vi "Test Get Keys from Map.vi"() -> ()   [LabVIEW 2020]
uses:
  5e20b283-b98d-45fe-82f2-655b53224886.vi
  <vilib>/addons/_JKI Toolkits/Caraya/classes/Assert/Assert Equal Value and Type_Variant.vi
  <vilib>/addons/_JKI Toolkits/Caraya/classes/Test/Test.lvclass
  <vilib>/addons/_JKI Toolkits/Caraya/classes/Assert/Assert.lvclass
panel:
  out "error out":errorcluster
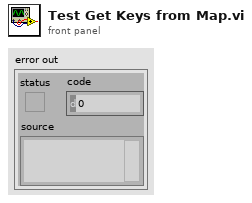
[diagram p1: front panel]
types:
  T1 = cluster{"Name":i32, "value":cluster{"bool":bool, "string":string}}[]
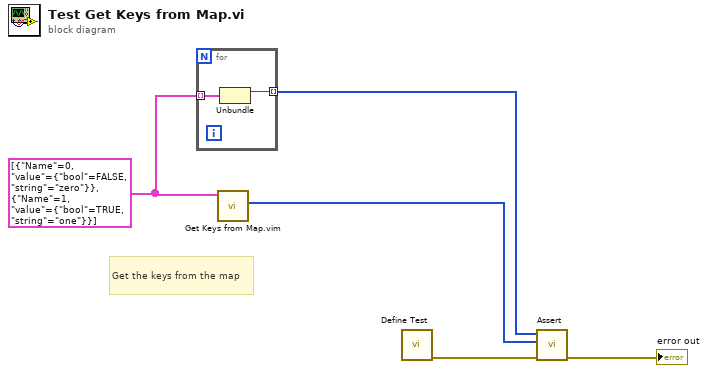
[diagram p0: block diagram]
diagram:
  w2 = T1 [{"Name"=0, "value"={"bool"=FALSE, "string"="zero"}}, {"Name"=1, "value"={"bool"=TRUE, "string"="one"}}] ("Array")
  # "Get the keys from the map"
  n1 = for {
    tunnel: w2 -> [w7] mode=indexing
    tunnel: [w6] -> w3 mode=indexing
    n2 = Unbundle(w7) -> ("Name"=w6:i32)  [unwired: 1 out]
  }
  n3 = call "Get Keys from Map.vim"("map"=w2) -> ("keys"=w1:i32[])  [unwired: 9 in, 1 out]
  n4 = call <vilib>:"Define Test.vi"() -> ("error out"=w5:errorcluster)  [unwired: 11 in]
  n5 = call-poly <vilib>:"Assert.vi"("error in (no error)"=w5, "Y"=w1, "X"=w3) -> ("error out"=→"error out":errorcluster)  [unwired: 8 in]
